vi "ReadFromFifo.vi"(8 "error in (no error)":errorcluster, 9 "Timeout (ms)":i32=5000, 10 "Number of Elements":u32, 11 "FpgaInterface in":refnum<class "FpgaInterface.lvclass">) -> (0 "error out":errorcluster, 1 "Elements Remaining":u32, 2 "Data":u32[](array[numeric]), 3 "FpgaInterface out":refnum<class "FpgaInterface.lvclass">)   [LabVIEW 2017, in "FpgaInterface.lvclass"]
uses:
  FpgaInterface.lvclass
  FpgaInterface.lvclass/FpgaInterface.ctl
  <vilib>/Utility/error.llb/Error Cluster From Error Code.vi
  <vilib>/rvi/errors/niLvFpgaAdjustHostInterfaceError.vi
  <vilib>/rvi/interface/nirviMethod/nirviMethod.xnode
  <vilib>/FPGAPlugInAG/Dynamic/niLvFpga_ReadFifo_Dynamic.vi
  <vilib>/rvi/errors/niLvFpgaMergeErrorWithErrorCode.vi
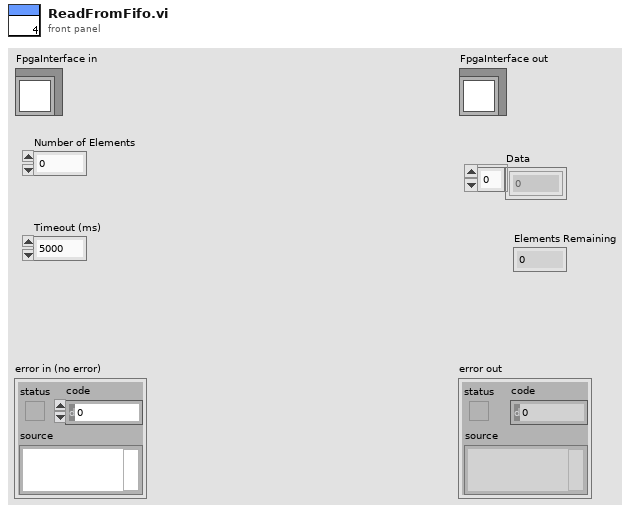
[diagram p1: front panel]
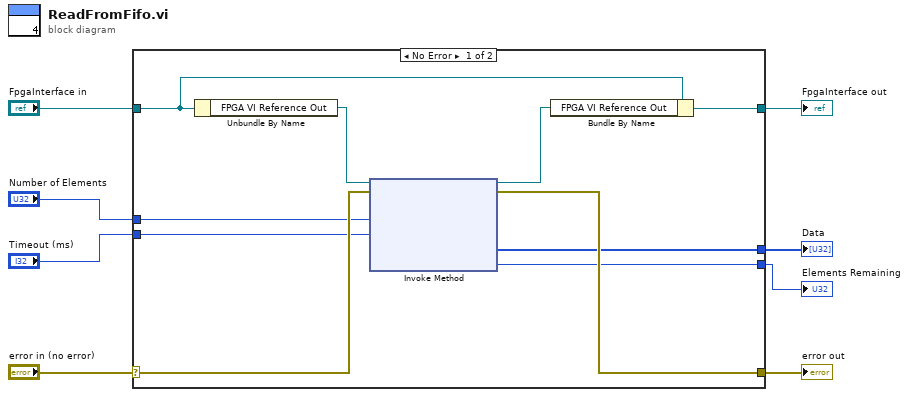
[diagram p0: block diagram]
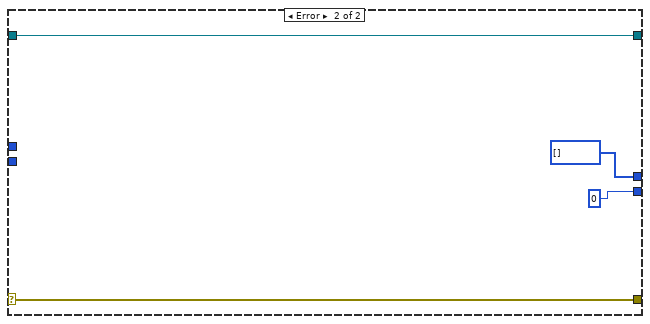
[diagram p2: hidden frame]
diagram:
  n1 = case shown="No Error" "error in (no error)" {
    selector: "error in (no error)" -> [w14 w22]
    tunnel: [w13 w22] -> w7
    tunnel: [w15 w21] -> w5
    tunnel: "FpgaInterface in" -> [w16 w21]
    tunnel: "Number of Elements" -> [w12 _]
    tunnel: "Timeout (ms)" -> [w11 _]
    tunnel: [w10 u32[] [] ("Data")] -> w2
    tunnel: [w9 u32 0 ("Elements Remaining")] -> w1
    frame No Error {
      n2 = Unbundle By Name(w16) -> ("FPGA VI Reference Out"=w18:refnum<k20>)
      n3 = xnode "Invoke Method"("FPGA VI Reference In"=w18, "error in"=w14, "Number of Elements"=w12, "Timeout (ms)"=w11) -> ("FPGA VI Reference Out"=w17:refnum<k20>, "error out"=w13:errorcluster, "Data"=w10:u32[], "Elements Remaining"=w9:u32)
      n4 = Bundle By Name(cluster=w16, "FPGA VI Reference Out"=w17) -> (w15:refnum<class "FpgaInterface.lvclass">)
    }
    frame Error {
    }
  }
  "error out" <- w7
  "FpgaInterface out" <- w5
  "Data" <- w2
  "Elements Remaining" <- w1
